vi "Payload_to_Macid.vi"(11 "ReadPayload":u8[](array[numeric])=[180, 119, 69, 76, 150, 124]) -> (3 "substring":string)   [LabVIEW 2024, in "Test_2.lvlib"]
uses:
  Test_2.lvlib
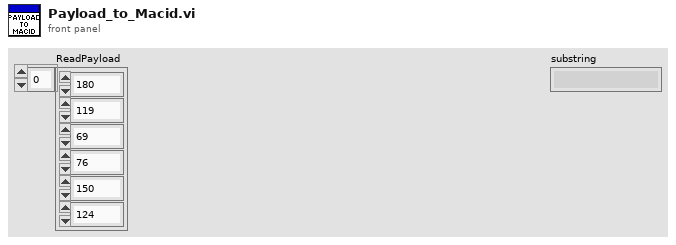
[diagram p1: front panel]
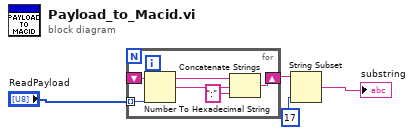
[diagram p0: block diagram]
diagram:
  n1 = for {
    tunnel: "ReadPayload" -> [w9] mode=indexing
    shift-right: [w6] -> w3
    shift-left: _ -> [w5]
    n2 = Number To Hexadecimal String(2:w9) -> (0:w8:string)  [unwired: 1 in]
    n3 = Concatenate Strings(w5, w8, ":" ("string")) -> (w6:string)
  }
  n4 = String Subset(string=w3, length (rest)=17 ("length (rest)")) -> (substring=→"substring":string)  [unwired: 1 in]
